vi "OpenMUXSession.vi"(8 "error in (no error)":errorcluster, 10 "gRPCid":T2, 11 "ctet_mux in":T1) -> (0 "error out":errorcluster, 3 "ctet_mux out":T1)   [LabVIEW 2019, in "ctet_mux_User Library.lvlib"]
uses:
  ctet_mux_User Library.lvlib
  Servers/ctet_mux/gRPC lvSupport/Server API/typeDefs/grpcId.ctl
  Types/ctet_mux.ctl
  Servers/ctet_mux/ctet_mux Class/RPC Messages/measurementservice_MUXOpenSessionResponse/measurementservice_MUXOpenSessionResponse_Data.ctl
  Servers/ctet_mux/ctet_mux Class/RPC Messages/measurementservice_ErrorOut/measurementservice_ErrorOut_Data.ctl
  Types/Switch Action.ctl
  Servers/ctet_mux/ctet_mux Class/ctet_mux.lvclass
  Servers/ctet_mux/gRPC lvSupport/gprc-lvsupport.lvlib
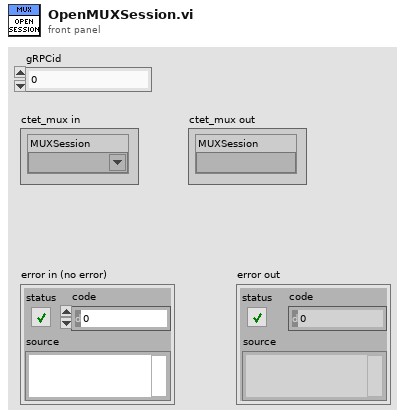
[diagram p1: front panel]
types:
  T1 = typedef "ctet_mux_User Library.lvlib/ctet_mux.ctl" = cluster{"MUXSession":refnum<k15>}
  T2 = typedef "ctet_mux.lvlib/gprc-lvsupport.lvlib/grpcId.ctl" = u64
  T3 = typedef "ctet_mux_User Library.lvlib/Switch Action.ctl" = enum16{"Get Switch State", "Initialize", "Connect Channel", "Open Channel", "Close Relay", "Open Relay", "Disconnect/Open All"}
  T4 = typedef "ctet_mux.lvlib/ctet_mux.lvclass/measurementservice_ErrorOut_Data.ctl" = cluster{"errCode":i64, "errMessage":string}
  T5 = typedef "ctet_mux.lvlib/ctet_mux.lvclass/measurementservice_MUXOpenSessionResponse_Data.ctl" = cluster{"error":T4}
  T6 = typedef "ctet_mux.lvlib/ctet_mux.lvclass/measurementservice_MUXOpenSessionRequest_Data.ctl" = cluster{"MUXName":string, "MUXTopology":string}
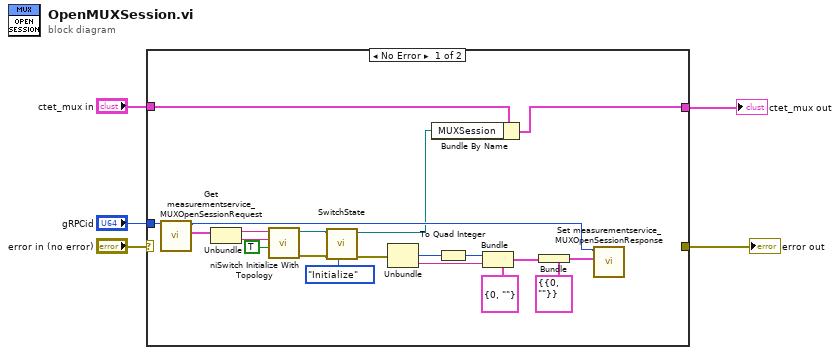
[diagram p0: block diagram]
diagram:
  n1 = case shown="No Error" "error in (no error)" {
    selector: "error in (no error)" -> [_ w27]
    tunnel: [_ w27] -> w5
    tunnel: "gRPCid" -> [w25 _]
    tunnel: "ctet_mux in" -> [w20 w26]
    tunnel: [w11 w26] -> w1
    frame No Error {
      n2 = call "Get measurementservice_MUXOpenSessionRequest.vi"("gRPCid"=w25) -> ("Message Data"=w24:T6, "gRPCid out"=w19:T2)  [unwired: 8 in, 1 out]
      n3 = Unbundle(w24) -> ("MUXName"=w23:string, "MUXTopology"=w22:string)
      n4 = call <instrlib>:"niSwitch Initialize With Topology.vi"("reset device (boolean value)"=TRUE, "topology name"=w22, "resource name"=w23) -> ("error out"=w9:errorcluster, "instrument handle out"=w10:refnum<k15>)  [unwired: 7 in]
      n5 = call "SwitchState.vi"("Switch Action"=Switch_Action."Initialize", "error in (no error)"=w9, "Switch Session"=w10) -> ("error out"=w7:errorcluster, "Switch Session out"=w8:refnum<k15>)  [unwired: 6 in, 1 out]
      n6 = Unbundle(w7) -> ("code"=w13:i32, "source"=w14:string)  [unwired: 1 out]
      n7 = Bundle By Name(cluster=w20, "MUXSession"=w8) -> (w11:T1)
      n8 = To Quad Integer(1:w13) -> (0:w12:i64)
      n9 = Bundle(cluster=T4 {"errCode"=0, "errMessage"=""} ("error"), "errCode"=w12, "errMessage"=w14) -> (w15:T4)
      n10 = Bundle(cluster=T5 {"error"={"errCode"=0, "errMessage"=""}} ("measurementservice_MUXOpenSessionResponse_Data"), "error"=w15) -> (w17:T5)
      n11 = call "Set measurementservice_MUXOpenSessionResponse.vi"("Message Data"=w17, "gRPCid"=w19) -> ()  [unwired: 9 in, 1 out]
    }
    frame Error {
    }
  }
  "error out" <- w5
  "ctet_mux out" <- w1
